vi "Write roomNumber.vi"(8 "error in (no error)":errorcluster, 10 "roomNumber":i32, 11 "Room":refnum<class "Room.lvclass">) -> (0 "error out":errorcluster, 3 "Room":refnum<class "Room.lvclass">)   [LabVIEW 2020, in "Room.lvclass"]
uses:
  Room.lvclass
  Room.lvclass/Room.ctl
  TypeDef/privateDataDVR.ctl
  TypeDef/privateData.ctl
  MazeSite/MazeSite.lvclass
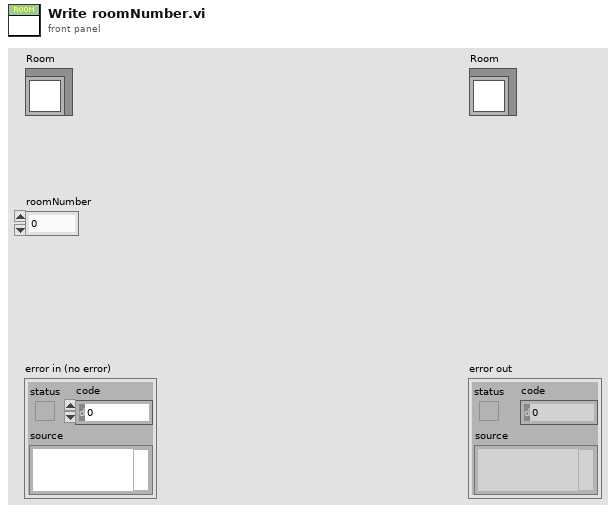
[diagram p1: front panel]
types:
  T1 = typedef "Room.lvclass/privateDataDVR.ctl" = refnum<data-value>
  T2 = typedef "Room.lvclass/privateData.ctl" = cluster{"sides":refnum<class "MazeSite.lvclass">[], "roomNumber":i32}
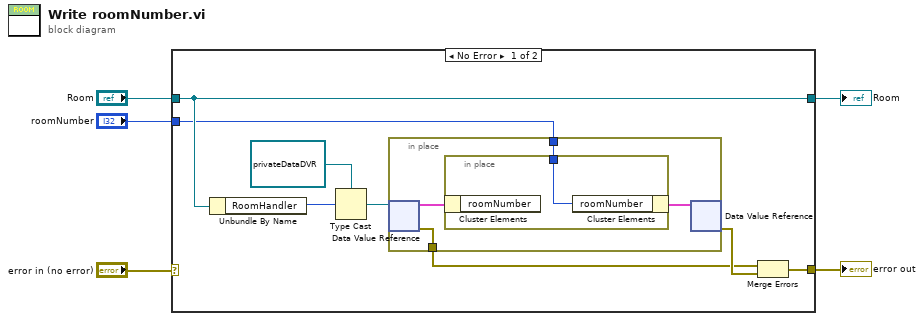
[diagram p0: block diagram]
diagram:
  n1 = case shown="No Error" "error in (no error)" {
    selector: "error in (no error)" -> [_ w19]
    tunnel: "Room" -> [w9 w20]
    tunnel: [w9 w20] -> w4
    tunnel: [w8 w19] -> w3
    tunnel: "roomNumber" -> [w6 _]
    frame No Error {
      n2 = Unbundle By Name(w9) -> ("RoomHandler"=w11:u32)
      n3 = Type Cast(type=T1 refnum ("privateDataDVR"), x=w11) -> (*(type *) &x=w13:T1)
      n4 = in-place {
        in-place-border: [w16] -> w10
        in-place-border: w6 -> [w15]
        n5 = in-place-dvr #1(w13) -> (w17:T2, w16:errorcluster)
        n6 = in-place {
          in-place-border: w15 -> [w18]
          n7 = in-place-cluster #2(w17) -> ()  [unwired: 1 out]
          n8 = in-place-cluster #2("roomNumber"=w18) -> (w14:T2)
        }
        n9 = in-place-dvr #1(w14) -> (w12:errorcluster)  [unwired: 1 out]
      }
      n10 = Merge Errors(w10, w12) -> (w8:errorcluster)
    }
    frame Error {
    }
  }
  "error out" <- w3
  "Room" <- w4
